vi "S1500_S7Com_REQ(SubVI).vi"(3 "Write Data":T8, 4 "Sequence#":u16, 5 "RW_CMD":T2={"Read Length"=1, "Data Block #"=1, "S7_Add_Area"=132, "Start Address"=0, "S7_Transport_Size"=3, "S7_Function"=4, "IP-Address"=""} {"S7_Function" items=["Read"=4, "Write"=5]; "S7_Transport_Size" items=["BIT"=1, "BYTE"=2, "CHAR"=3, "WORD"=4, "INT"=5, "DWORD"=6, "DINT"=7, "REAL"=8]; "S7_Add_Area" items=["P Area"=128, "I Area"=129, "O Area"=130, "M Area"=131, "DB Area"=132, "Counter"=40, "Timer"=41]}) -> (0 "Out Data":T6 format="X%02x", 2 "S7_Transport_Size":T1 items=["BIT"=1, "BYTE"=2, "CHAR"=3, "WORD"=4, "INT"=5, "DWORD"=6, "DINT"=7, "REAL"=8])   [LabVIEW 2018]
doc: "Forms the S7 Protocol Data Request."
uses:
  S1500_S7Com_Data_Array.ctl
  S1500_test_S7Com_HexByteArray.ctl
  S1500_S7Com_HexByte.ctl
  S1500_S7Com_RW_CMD.ctl
  S1500_S7Com_Address_Area.ctl
  S1500_S7Com_Start_Add.ctl
  S1500_S7Com_Transport_Size.ctl
  S1500_S7Com_Function.ctl
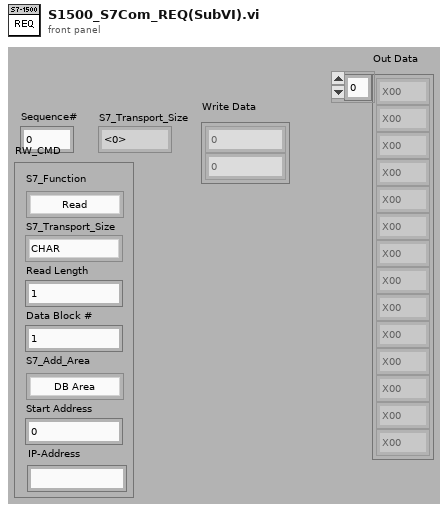
[diagram p1: front panel]
types:
  T1 = typedef "S1500_S7Com_Transport_Size.ctl" = u8
  T2 = typedef "S1500_S7Com_RW_CMD.ctl" = cluster{"Read Length":u16, "Data Block #":u16, "S7_Add_Area":T3, "Start Address":T4, "S7_Transport_Size":T1, "S7_Function":T5, "IP-Address":string}
  T3 = typedef "S1500_S7Com_Address_Area.ctl" = u8
  T4 = typedef "S1500_S7Com_Start_Add.ctl" = u16
  T5 = typedef "S1500_S7Com_Function.ctl" = u8
  T6 = typedef "S1500_test_S7Com_HexByteArray.ctl" = T7[]
  T7 = typedef "S1500_S7Com_HexByte.ctl" = u8
  T8 = typedef "S1500_S7Com_Data_Array.ctl" = i32[]
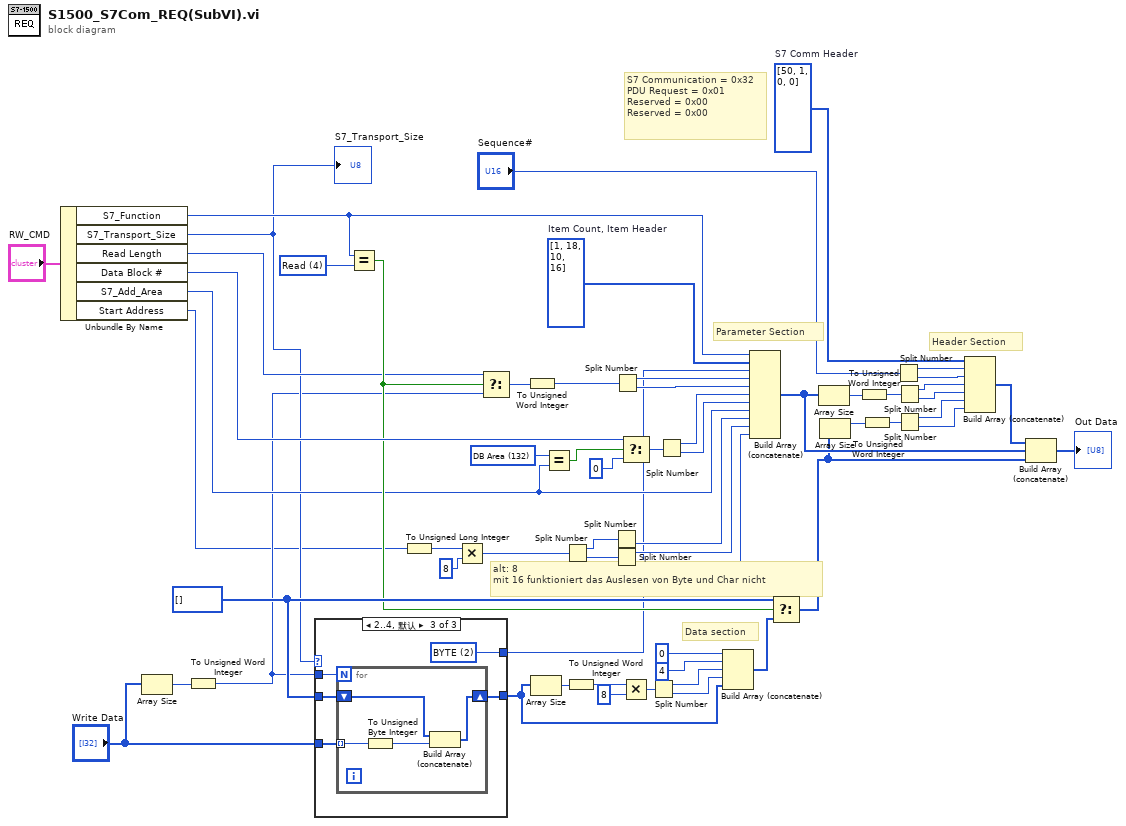
[diagram p0: block diagram]
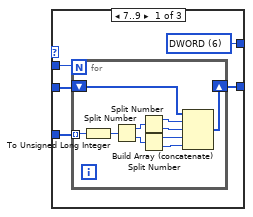
[diagram p2: hidden frame]
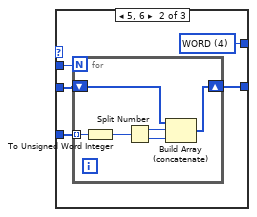
[diagram p3: hidden frame]
diagram:
  w16 = T6 [] ("S7_HexByte_Array")
  w27 = T5 4 items=["Read"=4, "Write"=5] ("S7_Function")
  w52 = T3 132 items=["P Area"=128, "I Area"=129, "O Area"=130, "M Area"=131, "DB Area"=132, "Counter"=40, "Timer"=41] ("S7_Add_Area")
  w34 = u8[] [1, 18, 10, 16]  # Item Count, Item Header
  w58 = u8[] [50, 1, 0, 0]  # S7 Comm Header
  # "alt: 8\nmit 16 funktioniert das Auslesen von Byte und Char nicht"
  # "Header Section"
  # "Parameter Section"
  # "Data section"
  # "S7 Communication = 0x32\nPDU Request = 0x01\nReserved = 0x00\nReserved = 0x00"
  n1 = Unbundle By Name("RW_CMD") -> ("S7_Function"=w14:T5, "S7_Transport_Size"=w6:T1, "Read Length"=w10:u16, "Data Block #"=w13:u16, "S7_Add_Area"=w9:T3, "Start Address"=w2:T4)
  "S7_Transport_Size" <- w6
  n2 = Array Size(array="Write Data") -> (size(s)=w8:i32)
  n3 = To Unsigned Word Integer(number=w8) -> (unsigned 16bit integer=w5:u16)
  n4 = case shown="2..4, 默认" w6 {
    tunnel: [w64 w79 w90] -> w18
    tunnel: "Write Data" -> [w63 w78 w88]
    tunnel: w16 -> [w62 w77 w89]
    tunnel: w5 -> [w61 w76 w87]
    tunnel: [w60 w75 w86] -> w1
    frame 7..9 {
      w60 = T1 6 items=["BIT"=1, "BYTE"=2, "CHAR"=3, "WORD"=4, "INT"=5, "DWORD"=6, "DINT"=7, "REAL"=8] ("S7_Transport_Size")
      n5 = for {
        N: w61 -> [_]
        tunnel: w63 -> [w66] mode=indexing
        shift-right: [w74] -> w64
        shift-left: w62 -> [w65]
        n6 = To Unsigned Long Integer(number=w66) -> (unsigned 32bit integer=w67:u32)
        n7 = Split Number(x=w67) -> (hi(x)=w73:u16, lo(x)=w72:u16)
        n8 = Split Number(x=w73) -> (hi(x)=w71:u8, lo(x)=w70:u8)
        n9 = Split Number(x=w72) -> (hi(x)=w68:u8, lo(x)=w69:u8)
        n10 = Build Array (concatenate)(w65, w71, w70, w68, w69) -> (w74:T6)
      }
    }
    frame 5, 6 {
      w75 = T1 4 items=["BIT"=1, "BYTE"=2, "CHAR"=3, "WORD"=4, "INT"=5, "DWORD"=6, "DINT"=7, "REAL"=8] ("S7_Transport_Size")
      n11 = for {
        N: w76 -> [_]
        tunnel: w78 -> [w81] mode=indexing
        shift-right: [w85] -> w79
        shift-left: w77 -> [w80]
        n12 = To Unsigned Word Integer(number=w81) -> (unsigned 16bit integer=w82:u16)
        n13 = Split Number(x=w82) -> (hi(x)=w84:u8, lo(x)=w83:u8)
        n14 = Build Array (concatenate)(w80, w84, w83) -> (w85:T6)
      }
    }
    frame 2..4, Default {
      w86 = T1 2 items=["BIT"=1, "BYTE"=2, "CHAR"=3, "WORD"=4, "INT"=5, "DWORD"=6, "DINT"=7, "REAL"=8] ("S7_Transport_Size")
      n15 = for {
        N: w87 -> [_]
        shift-right: [w94] -> w90
        shift-left: w89 -> [w93]
        tunnel: w88 -> [w92] mode=indexing
        n16 = To Unsigned Byte Integer(number=w92) -> (unsigned 8bit integer=w91:u8)
        n17 = Build Array (concatenate)(w93, w91) -> (w94:T6)
      }
    }
  }
  n18 = Equal?(x=w14, y=w27) -> (x = y?=w12:bool)
  n19 = To Unsigned Long Integer(number=w2) -> (unsigned 32bit integer=w4:u32)
  n20 = Multiply(x=w4, y=T4 8) -> (x*y=w3:u32)
  n21 = Select(t=w10, s=w12, f=w5) -> (s? t:f=w11:u16)
  n22 = To Unsigned Word Integer(number=w11) -> (unsigned 16bit integer=w7:u16)
  n23 = Array Size(array=w18) -> (size(s)=w49:i32)
  n24 = Equal?(x=w52, y=w9) -> (x = y?=w53:bool)
  n25 = Split Number(x=w3) -> (hi(x)=w36:u16, lo(x)=w35:u16)
  n26 = To Unsigned Word Integer(number=w49) -> (unsigned 16bit integer=w19:u16)
  n27 = Split Number(x=w36) -> (lo(x)=w22:u8)  [unwired: 1 out]
  n28 = Split Number(x=w35) -> (hi(x)=w23:u8, lo(x)=w24:u8)
  n29 = Split Number(x=w7) -> (hi(x)=w31:u8, lo(x)=w32:u8)
  n30 = Select(t=w13, s=w53, f=u16 0) -> (s? t:f=w56:u16)
  n31 = Multiply(x=w19, y=u16 8) -> (x*y=w20:u16)
  n32 = Split Number(x=w20) -> (hi(x)=w46:u8, lo(x)=w45:u8)
  n33 = Split Number(x=w56) -> (hi(x)=w55:u8, lo(x)=w54:u8)
  n34 = Build Array (concatenate)(u8 0, u8 4, w46, w45, w18) -> (w25:T6)
  n35 = Build Array (concatenate)(w14, w34, w1, w31, w32, w55, w54, w9, w22, w23, w24) -> (w29:T3[])
  n36 = Select(t=w16, s=w12, f=w25) -> (s? t:f=w26:T6)
  n37 = Array Size(array=w29) -> (size(s)=w33:i32)
  n38 = Array Size(array=w26) -> (size(s)=w44:i32)
  n39 = To Unsigned Word Integer(number=w33) -> (unsigned 16bit integer=w41:u16)
  n40 = To Unsigned Word Integer(number=w44) -> (unsigned 16bit integer=w38:u16)
  n41 = Split Number(x="Sequence#") -> (hi(x)=w51:u8, lo(x)=w50:u8)
  n42 = Split Number(x=w41) -> (hi(x)=w43:u8, lo(x)=w42:u8)
  n43 = Split Number(x=w38) -> (hi(x)=w40:u8, lo(x)=w39:u8)
  n44 = Build Array (concatenate)(w58, w51, w50, w43, w42, w40, w39) -> (w30:u8[])
  n45 = Build Array (concatenate)(w30, w29, w26) -> (→"Out Data":T6)
